vi "Write value as Numeric.vi"(8 "error in (no error)":errorcluster, 10 "value":dbl, 11 "JSON Value in":refnum<class "JSON Value.lvclass">) -> (0 "error out":errorcluster, 3 "JSON Value out":refnum<class "JSON Value.lvclass">)   [LabVIEW 2016, in "JSON Value.lvclass"]
uses:
  JSON Value.lvclass
  JSON Value.lvclass/JSON Value.ctl
  JSON Types.ctl
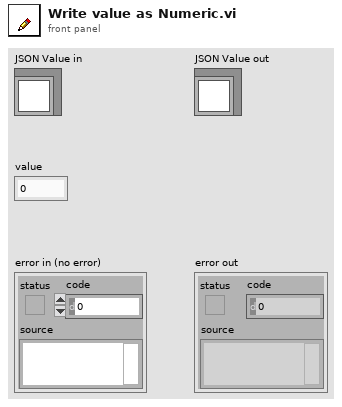
[diagram p1: front panel]
types:
  T1 = typedef "JSON Value.lvclass/JSON Types.ctl" = enum8{"String", "Numeric", "Boolean", "NULL", "Object", "Array"}
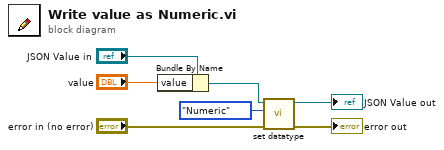
[diagram p0: block diagram]
diagram:
  n1 = Bundle By Name(cluster="JSON Value in", "value"="value") -> (w2:refnum<class "JSON Value.lvclass">)
  n2 = call "set datatype.vi"("error in (no error)"="error in (no error)", "datatype"=JSON_Types."Numeric", "JSON Helper in"=w2) -> ("error out"=→"error out":errorcluster, "JSON Helper out"=→"JSON Value out":refnum<class "JSON Value.lvclass">)  [unwired: 7 in]
